vi "create default alias.vi"(8 "error in":errorcluster, 11 "configuration in":refnum<class "NISE_CEF_serializable node folder configuration.lvclass">) -> (0 "error out":errorcluster, 2 "default alias":string, 3 "configuration out":refnum<class "NISE_CEF_serializable node folder configuration.lvclass">)   [LabVIEW 2013, in "NISE_CEF_serializable node folder configuration.lvclass"]
uses:
  NISE_CEF_serializable node folder configuration.lvclass
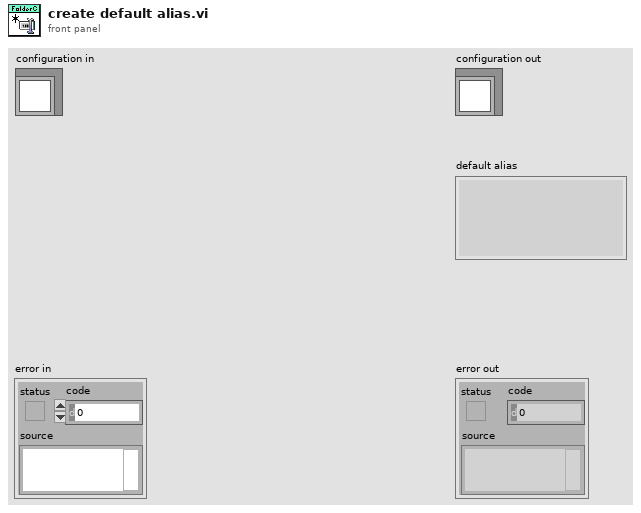
[diagram p1: front panel]
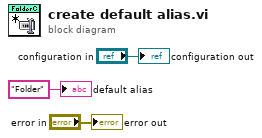
[diagram p0: block diagram]
diagram:
  "error out" <- "error in"
  "configuration out" <- "configuration in"
  "default alias" <- "Folder" ("default alias")
